vi "Test Process Error Caused by Request in Process is Handled.vi"(8 "error in (no error)":errorcluster, 11 "Process Test In":refnum<class "Process Dev Test.lvclass">) -> (0 "error out":errorcluster, 3 "Process Test Out":refnum<class "Process Dev Test.lvclass">)   [LabVIEW 2020, in "Process Dev Test.lvclass"]
uses:
  Process Dev Test.lvclass
  C:/Program Files (x86)/National Instruments/LabVIEW 2020/vi.lib/Astemes/LUnit/Test Case.lvclass
  source/Framework Test Suite/Mock Process/Mock Process.lvclass
  C:/git/astemes-triarc-framework/source/Framework/Process/Process.lvclass
  source/Framework Test Suite/Mock Error Handler/Mock Error Handler.lvclass
  C:/git/astemes-triarc-framework/source/Framework/Error Handler Interface/Error Handler Interface.lvclass
  source/Framework/Process/Process.lvclass/Process.ctl
  <vilib>/Astemes/LUnit/Test Case.lvclass/Test Case.ctl
  46d70d04-9be4-4580-a401-07f2d837d1b6.vi
  source/Framework/Process/Protected/Messaging/Send Message.vi
  source/Framework/Process/Public/Lifecycle/Get Lifecycle State.vi
  source/Framework/Process/Protected/SubVIs/Set Context.vi
  source/Framework/Process/Private/SubVIs/Wait for finish.vi
  source/Framework/Process/Private/SubVIs/Set Lifecycle State.vi
  <vilib>/Astemes/LUnit/Append Pass Result.vi
  <vilib>/Astemes/LUnit/Append Fail Result.vi
  <vilib>/Astemes/LUnit/Describe Comparison.vi
  <vilib>/Astemes/LUnit/Compare Variants.vi
  source/Framework/Process/Private/SubVIs/Handle Debug Data.vi
  <vilib>/Astemes/LUnit/Variant to string.vi
  source/Framework/Logging/Log Debug.vi
  <vilib>/AdvancedString/1D String Array to Delimited String.vi
  <vilib>/Utility/High Resolution Relative Seconds.vi
  <vilib>/Utility/error.llb/Error Cluster From Error Code.vi
  source/Framework/Process/Public/Read Name.vi
  <vilib>/Utility/Data Type/Get Type Information.vi
  <vilib>/Utility/LVClass/Get LV Class Name.vi
  source/Framework/Process/Process.lvclass
  source/Framework/Callback/Callback.lvclass
  <vilib>/ErrorRing/Error Ring.xnode
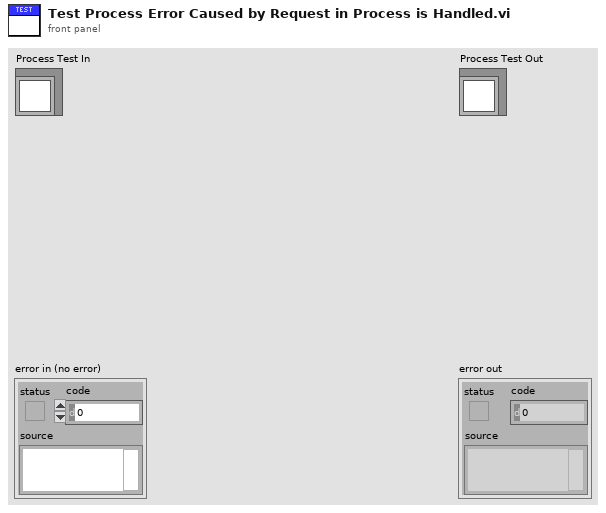
[diagram p1: front panel]
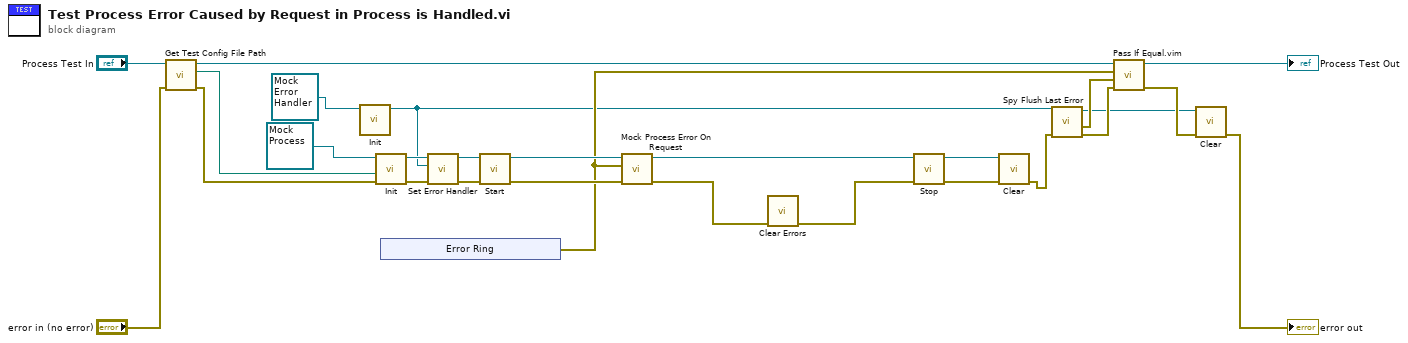
[diagram p0: block diagram]
diagram:
  n1 = call "Get Test Config File Path.vi"("error in (no error)"="error in (no error)", "Process Test In"="Process Test In") -> ("error out"=w22:errorcluster, "Test config path"=w23:path, "Process Test Out"=w16:refnum<class "Process Dev Test.lvclass">)  [unwired: 7 in]
  n2 = call-dynamic "Init.vi"("Mock Error Handler In"=refnum<class "Mock Error Handler.lvclass"> refnum) -> ("Mock Error Handler Out"=w1:refnum<class "Mock Error Handler.lvclass">)  [unwired: 9 in, 1 out]
  n3 = call-dynamic "Init.vi"("error in (no error)"=w22, "Config File Path"=w23, "Mock Process In"=refnum<class "Mock Process.lvclass"> refnum ("Mock Process.lvclass")) -> ("error out"=w25:errorcluster, "Mock Process Out"=w11:refnum<class "Mock Process.lvclass">)  [unwired: 7 in]
  n4 = xnode "Error Ring"() -> ("error out"=w7:errorcluster)
  n5 = call "Set Error Handler.vi"("error in (no error)"=w25, "Error Handler"=w1, "Process In"=w11) -> ("error out"=w12:errorcluster, "Process Out"=w10:refnum<class "Mock Process.lvclass">)  [unwired: 7 in]
  n6 = call "Start.vi"("error in (no error)"=w12, "Process In"=w10) -> ("error out"=w20:errorcluster, "Process Out"=w18:refnum<class "Mock Process.lvclass">)  [unwired: 7 in, 1 out]
  n7 = call "Mock Process Error On Request.vi"("error in (no error)"=w20, "Mock Error"=w7, "Mock Process in"=w18) -> ("error out"=w14:errorcluster, "Mock Process out"=w17:refnum<class "Mock Process.lvclass">)  [unwired: 6 in, 1 out]
  n8 = call <vilib>:"Clear Errors.vi"("error in (no error)"=w14) -> ("error out"=w13:errorcluster)  [unwired: 5 in, 1 out]
  n9 = call "Stop.vi"("error in (no error)"=w13, "Process In"=w17) -> ("error out"=w19:errorcluster, "Process Out"=w27:refnum<class "Mock Process.lvclass">)  [unwired: 7 in, 1 out]
  n10 = call-dynamic "Clear.vi"("error in (no error)"=w19, "Mock Process In"=w27) -> ("error out"=w6:errorcluster)  [unwired: 9 in]
  n11 = call "Spy Flush Last Error.vi"("error in (no error)"=w6, "Mock Error Handler In"=w1) -> ("error out"=w9:errorcluster, "Error"=w8:errorcluster, "Mock Error Handler Out"=w4:refnum<class "Mock Error Handler.lvclass">)  [unwired: 7 in]
  n12 = call "Pass If Equal.vim"("error in (no error)"=w9, "Actual"=w8, "Expected"=w7, "LUnit Test Case In"=w16) -> ("error out"=w5:errorcluster, "LUnit Test Case Out"=→"Process Test Out":refnum<class "Process Dev Test.lvclass">)  [unwired: 6 in]
  n13 = call-dynamic "Clear.vi"("error in (no error)"=w5, "Mock Process In"=w4) -> ("error out"=→"error out":errorcluster)  [unwired: 9 in]
